vi "LoadPartInfo.vi"() -> (0 "W/O Qty":string="20000", 1 "Date Code (YYWW) 2":string="1644" caption="D/C (YYWW)", 2 "Lot Number (6 digits) 2":string="123456" caption="L/N (6 digits)", 3 "Part Number_Die Ver_Field 2":string="206CAH" caption="P/N_Die Ver_Field", 4 "Work Order 2":string="1644" caption="Work Order", 5 "Operator 2":string="A1644" caption="Operator")   [LabVIEW 2013]
panel:
  in  "OK":bool
  in  "Operator":string="A1644"
  in  "W/O Qty":string="20000"
  in  "Work Order":string="1644"
  in  "Date Code (YYWW)":string="1644" caption="D/C (YYWW)"
  in  "Lot Number (6 digits)":string="123456" caption="L/N (6 digits)"
  in  "Part Number_Die Ver_Field":string="206CAH" caption="P/N_Die Ver_Field"
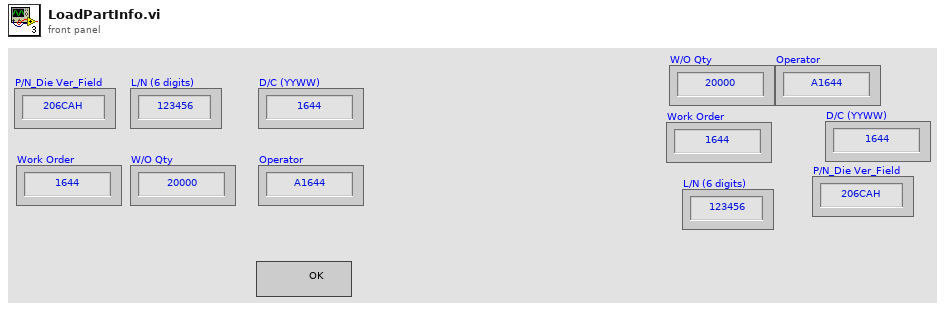
[diagram p1: front panel]
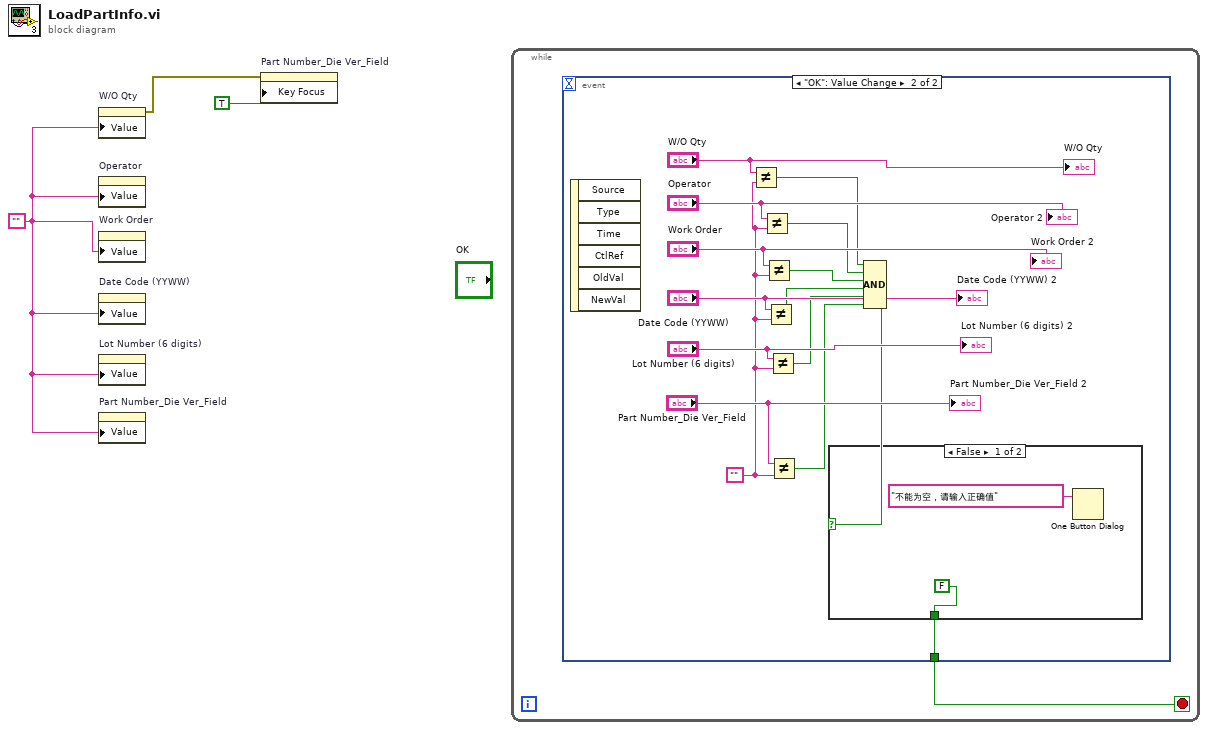
[diagram p0: block diagram]
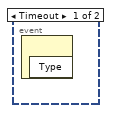
[diagram p2: hidden frame]
diagram:
  w3 = ""
  n1 = property on="W/O Qty" class="Str"("Value"=w3) -> (error out=w1:errorcluster)  [unwired: 2 in, 1 out]
  n2 = property on="Operator" class="Str"("Value"=w3) -> ()  [unwired: 2 in, 2 out]
  n3 = property on="Work Order" class="Str"("Value"=w3) -> ()  [unwired: 2 in, 2 out]
  n4 = property on="Date Code (YYWW)" class="Str"("Value"=w3) -> ()  [unwired: 2 in, 2 out]
  n5 = property on="Lot Number (6 digits)" class="Str"("Value"=w3) -> ()  [unwired: 2 in, 2 out]
  n6 = property on="Part Number_Die Ver_Field" class="Str"("Value"=w3) -> ()  [unwired: 2 in, 2 out]
  n7 = property on="Part Number_Die Ver_Field" class="Str"(error in=w1, "Key Focus"=TRUE) -> ()  [unwired: 1 in, 2 out]
  n8 = while {
    stop <- w4 stop-if-true
    n9 = event shown="[1] \"OK\": Value Change" {
      selector: _ -> [_ _]
      dyn-events: _ -> [_ _]
      timeout: _ -> [_ _]
      tunnel: [_ w5] -> w4
      event Timeout {
        n10 = event-data() -> ()  [unwired: 1 in, 1 out]
      }
      event "OK": Value Change {
        w13 = ""
        n11 = event-data() -> ()  [unwired: 1 in, 6 out]
        n12 = Not Equal?(x="W/O Qty", y=w13) -> (x != y?=w12:bool)
        n13 = Not Equal?(x="Operator", y=w13) -> (x != y?=w11:bool)
        n14 = Not Equal?(x="Work Order", y=w13) -> (x != y?=w10:bool)
        n15 = Not Equal?(x="Date Code (YYWW)", y=w13) -> (x != y?=w9:bool)
        n16 = Not Equal?(x="Lot Number (6 digits)", y=w13) -> (x != y?=w8:bool)
        n17 = Not Equal?(x="Part Number_Die Ver_Field", y=w13) -> (x != y?=w7:bool)
        n18 = Compound Arithmetic op=AND(w12, w11, w10, w9, w8, w7) -> (w6:bool)
        n19 = case shown="False" w6 {
          selector: w6 -> [_ w22]
          tunnel: [FALSE w22] -> w5
          frame False {
            n20 = One Button Dialog(message="不能为空，请输入正确值") -> ()  [unwired: 1 in, 1 out]
          }
          frame True {
          }
        }
        "W/O Qty" <- "W/O Qty"
        "Operator 2" <- "Operator"
        "Work Order 2" <- "Work Order"
        "Date Code (YYWW) 2" <- "Date Code (YYWW)"
        "Lot Number (6 digits) 2" <- "Lot Number (6 digits)"
        "Part Number_Die Ver_Field 2" <- "Part Number_Die Ver_Field"
      }
    }
  }
